vi "DataFileNode_Entry_V4.vi"(8 "error in (no error)":errorcluster, 10 "Queued Elements":T1, 11 "Byte Stream File in":refnum<file>) -> (0 "error out":errorcluster, 3 "Byte Stream File out":refnum<file>)   [LabVIEW 2019]
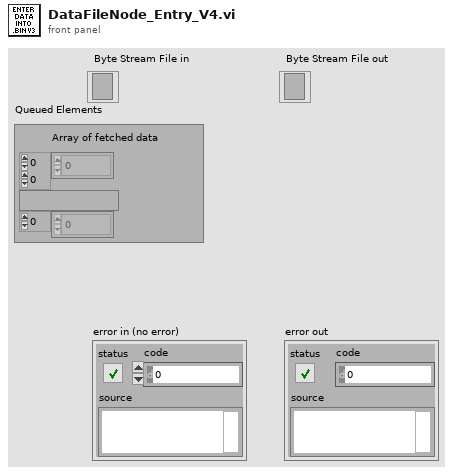
[diagram p1: front panel]
types:
  T1 = cluster{"Array of fetched data":dbl[][], string, i32[]}
  T2 = enum16{"big-endian, network order", "native, host order", "little-endian"}
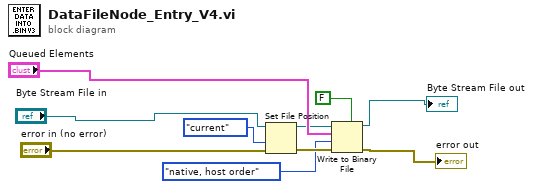
[diagram p0: block diagram]
diagram:
  n1 = Set File Position(refnum="Byte Stream File in", from (0:start)=enum16{"start", "end", "current"}."current", error in="error in (no error)") -> (refnum out=w4:refnum<file>, error out=w3:errorcluster)  [unwired: 1 in]
  n2 = Write to Binary File(file (use dialog)=w4, data="Queued Elements", error in=w3, 5:FALSE ("prepend array or string size? (T)"), 9:T2."native, host order" ("byte order (0:big-endian, network order)")) -> (refnum out=→"Byte Stream File out":refnum<file>, error out=→"error out":errorcluster)  [unwired: 1 in, 1 out]
